vi "Zykluszeit fuer Messwert Abfrage berechnen.vi"(8 "NoOfScan ALT":u32, 11 "NoOfScan NEU":u32) -> (0 "Zykluszeit ToolWeb":u32, 1 "Zykluszeit Messdatenverteiler":u32, 3 "NoOfScan":u32)   [LabVIEW 2020, in "FT-IR.lvlib"]
uses:
  FT-IR.lvlib
  Aktionen EVID-Codes.ctl
  AK interface/TCP Timeout Aktionen - FTIR.ctl
  AK interface/AK-Interface.lvlib
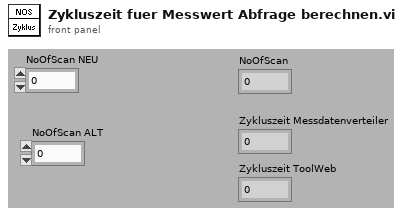
[diagram p1: front panel]
types:
  T1 = typedef "FT-IR.lvlib/Aktionen EVID-Codes.ctl" = enum16{"lesen", "setzen", "laden", "speichern", "1Hz/5Hz", "Smoothing", "Rolling Average"}
  T2 = typedef "FT-IR.lvlib/1Hz-5Hz Geraet.ctl" = u16
  T3 = typedef "FT-IR.lvlib/AK-Interface.lvlib/TCP Timeout Aktionen - FTIR.ctl" = enum16{"lesen", "setzen"}
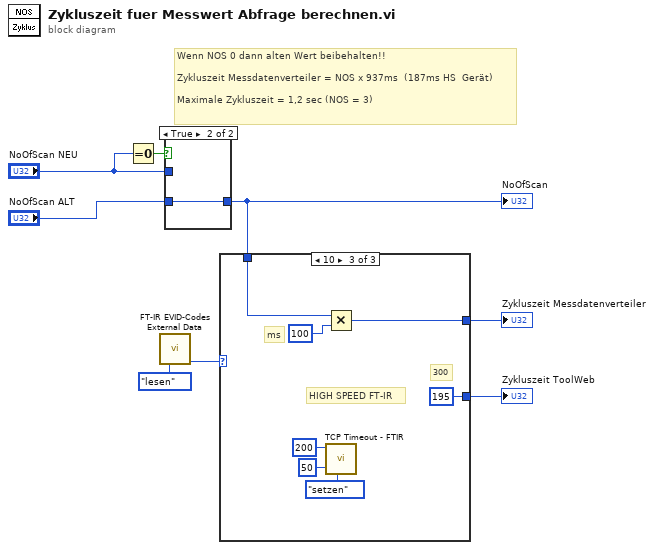
[diagram p0: block diagram]
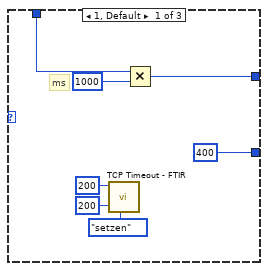
[diagram p2: hidden frame]
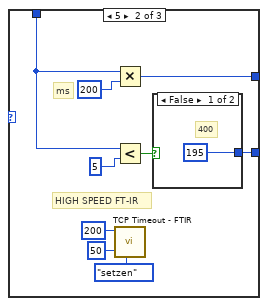
[diagram p3: hidden frame]
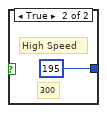
[diagram p4: hidden frame]
diagram:
  # "Wenn NOS 0 dann alten Wert beibehalten!!\n\nZykluszeit Messdatenverteiler = NOS x 937ms  (187ms HS  Gerät)\n\nMaximale Zykluszeit = 1,2 sec (NOS = 3)"
  n1 = Equal To 0?(x="NoOfScan NEU") -> (x = 0?=w8:bool)
  n2 = call "FT-IR EVID-Codes External Data.vi"("Aktionen"=Aktionen_EVID-Codes."lesen") -> ("1Hz/5Hz Gerät"=w1:T2)  [unwired: 9 in, 5 out]
  n3 = case shown="True" w8 {
    tunnel: "NoOfScan NEU" -> [w9 _]
    tunnel: "NoOfScan ALT" -> [_ w10]
    tunnel: [w9 w10] -> w3
    frame False {
    }
    frame True {
    }
  }
  "NoOfScan" <- w3
  n4 = case shown="10" w1 {
    tunnel: [w17 w22 w33] -> w5
    tunnel: [u32 400 ("Zykluszeit ToolWeb") w21 u32 195 ("Zykluszeit ToolWeb")] -> w4
    tunnel: w3 -> [w15 w26 w35]
    frame 1, Default {
      # "ms"
      n5 = call "TCP Timeout - FTIR.vi"("Aktionen Timeout"=TCP_Timeout_Aktionen_-_FTIR."setzen", "Timeout lesen"=200, "Timeout schreiben"=200) -> ()  [unwired: 7 in, 2 out]
      n6 = Multiply(x=w15, y=u32 1000) -> (x*y=w17:u32)
    }
    frame 5 {
      # "HIGH SPEED FT-IR"
      # "ms"
      n7 = Multiply(x=w26, y=u32 200) -> (x*y=w22:u32)
      n8 = Less?(x=w26, y=u32 5) -> (x < y?=w24:bool)
      n9 = call "TCP Timeout - FTIR.vi"("Aktionen Timeout"=TCP_Timeout_Aktionen_-_FTIR."setzen", "Timeout lesen"=50, "Timeout schreiben"=200) -> ()  [unwired: 7 in, 2 out]
      n10 = case shown="False" w24 {
        tunnel: [u32 195 ("Zykluszeit ToolWeb") u32 195 ("Zykluszeit ToolWeb")] -> w21
        frame False {
          # "400"
        }
        frame True {
          # "300"
          # "High Speed"
        }
      }
    }
    frame 10 {
      # "300"
      # "HIGH SPEED FT-IR"
      # "ms"
      n11 = Multiply(x=w35, y=u32 100) -> (x*y=w33:u32)
      n12 = call "TCP Timeout - FTIR.vi"("Aktionen Timeout"=TCP_Timeout_Aktionen_-_FTIR."setzen", "Timeout lesen"=50, "Timeout schreiben"=200) -> ()  [unwired: 7 in, 2 out]
    }
  }
  "Zykluszeit Messdatenverteiler" <- w5
  "Zykluszeit ToolWeb" <- w4
